vi "Hat Switch Interpreter.vi"(5 "JoystickDevRef":T1={"Device"=enum."USB 1"}) -> (0 "Buttons":bool[](array[boolean]), 1 "Buttons Pressed":bool[](array[boolean]), 2 "Enum Status":T4(ring), 3 "Numeric Status":u8, 4 "Hat Switch Cluster":T3)   [LabVIEW 2014]
uses:
  <vilib>/Rock Robotics/WPI/Joystick/WPI_JoystickDevRef.ctl
  <vilib>/Rock Robotics/WPI/Joystick/WPI_JoystickDeviceEnum.ctl
panel:
  # "ENUM LAYOUT"
  # "NUMERIC LAYOUT"
  # "North"
  # "1"
  # "Northeast"
  # "2"
  # "Northwest"
  # "8"
  # "West"
  # "East"
  # "7"
  # "3"
  # "Null"
  # "0"
  # "Southwest"
  # "Southeast"
  # "6"
  # "4"
  # "5"
  # "South"
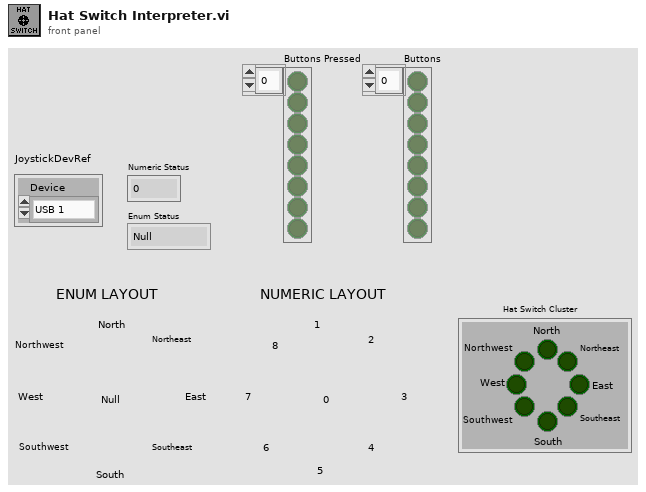
[diagram p1: front panel]
types:
  T1 = typedef "WPI_JoystickDevRef.ctl" = cluster{"Device":T2}
  T2 = typedef "WPI_JoystickDeviceEnum.ctl" = enum16{"USB 0", "USB 1", "USB 2", "USB 3", "USB 4", "USB 5"}
  T3 = cluster{"North":bool, "Northeast":bool, "East":bool, "Southeast":bool, "South":bool, "Southwest":bool, "West":bool, "Northwest":bool}
  T4 = enum8{"Null", "North", "Northeast", "East", "Southeast", "South", "Southwest", "West", "Northwest"}
  T5 = cluster{"North":bool, "Northeast":bool, "East":bool, "Southeast":bool, "South":bool, "Northwest":bool, "Southwest":bool, "West":bool}
  T6 = cluster{"[0]":bool, "[1]":bool, "[2]":bool, "[3]":bool, "[4]":bool, "[5]":bool, "[6]":bool, "[7]":bool, "[8]":bool}
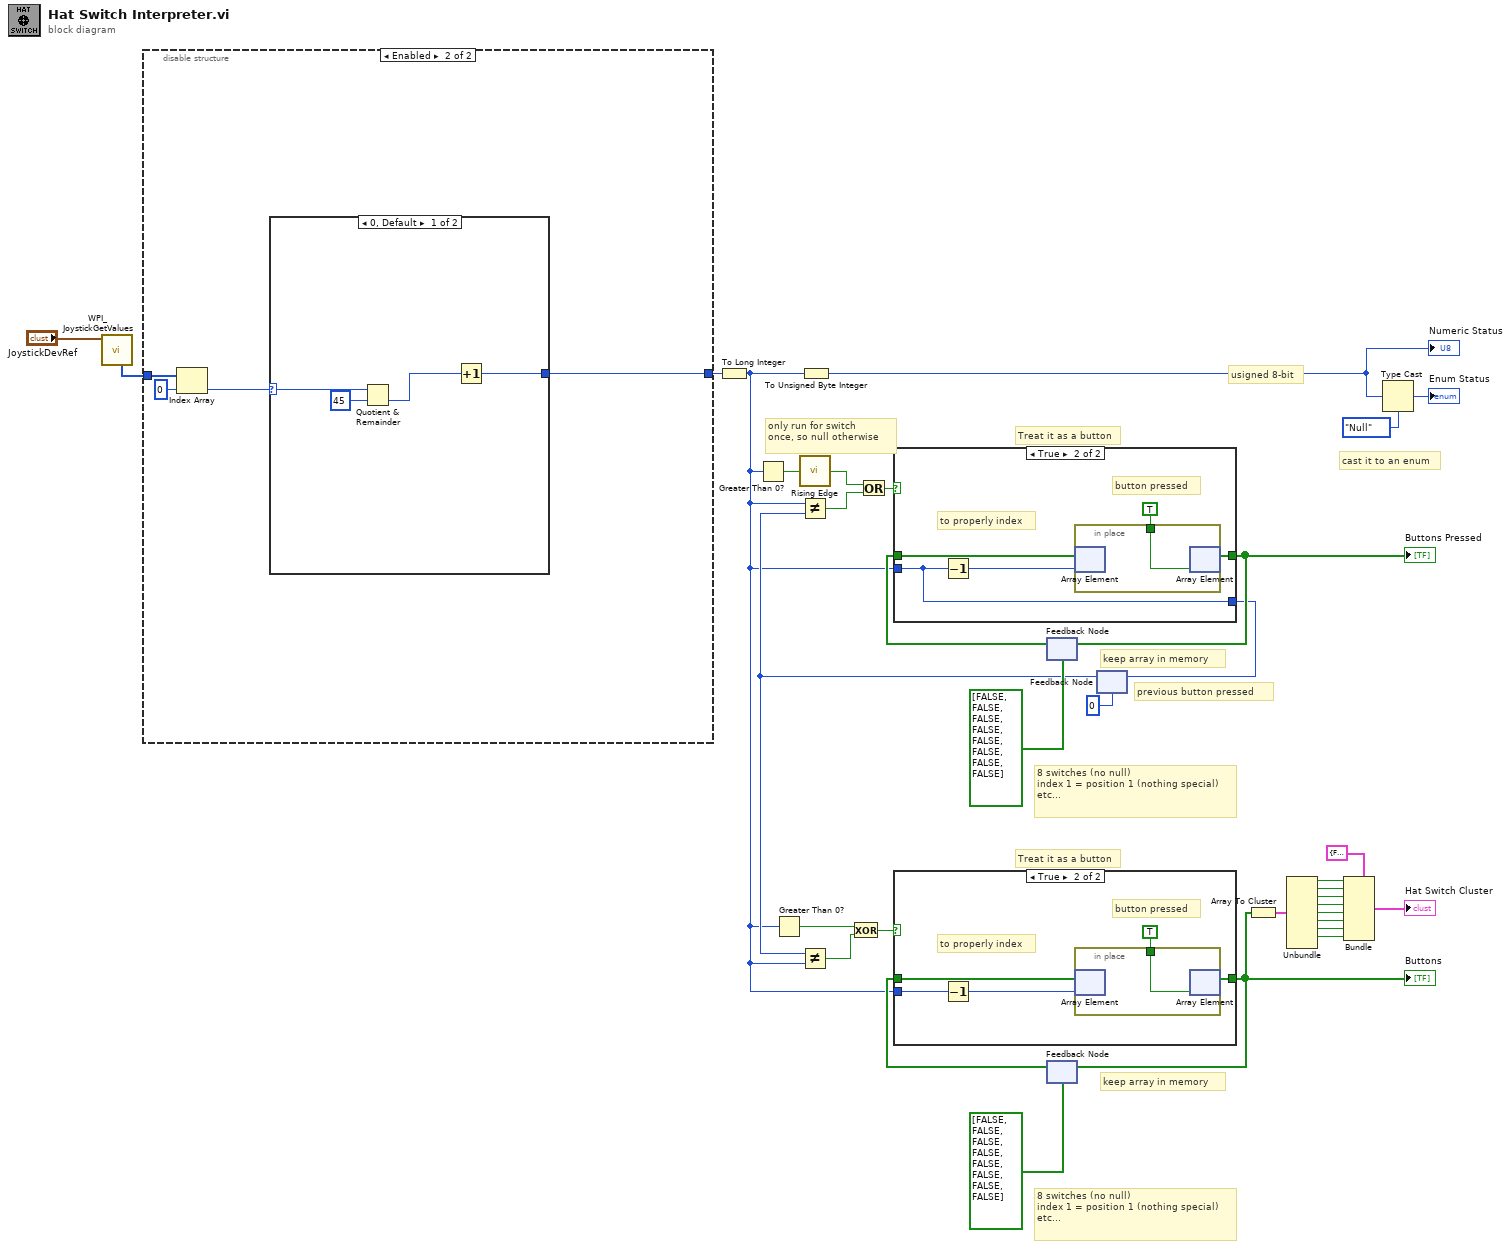
[diagram p0: block diagram]
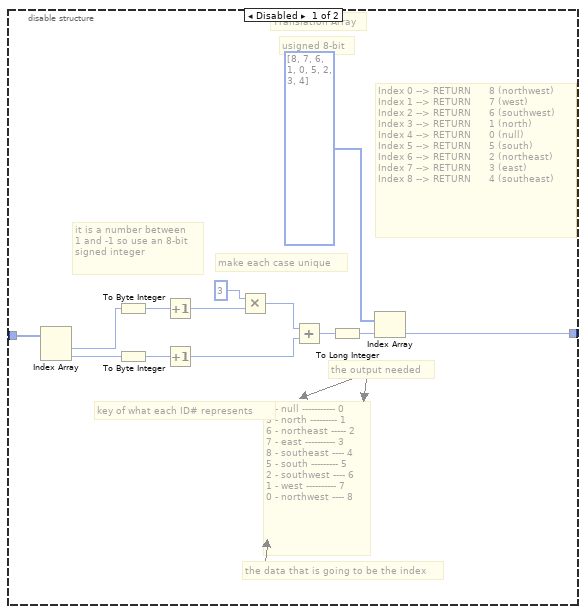
[diagram p2: hidden frame]
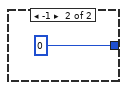
[diagram p3: hidden frame]
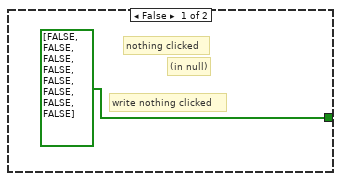
[diagram p4: hidden frame]
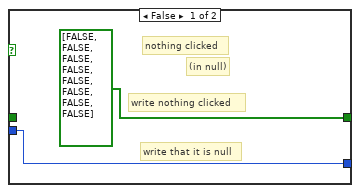
[diagram p5: hidden frame]
diagram:
  # "cast it to an enum"
  # "keep array in memory"
  # "8 switches (no null)\nindex 1 = position 1 (nothing special)\netc..."
  # "Treat it as a button"
  # "only run for switch\nonce, so null otherwise"
  # "keep array in memory"
  # "previous button pressed"
  # "8 switches (no null)\nindex 1 = position 1 (nothing special)\netc..."
  # "Treat it as a button"
  # "usigned 8-bit"
  n1 = call <vilib>:"WPI_JoystickGetValues.vi"("JoystickDevRef"="JoystickDevRef") -> ("POVs"=w4:i16[])  [unwired: 6 in, 4 out]
  n2 = disable-structure shown="Enabled" {
    disable-tunnel: [w38 w48] -> w26
    disable-tunnel: w4 -> [w37 w51]
    frame Disabled {
      # "usigned 8-bit"
      # "the data that is going to be the index"
      # "the output needed"
      # "key of what each ID# represents"
      # "Index 0 --> RETURN      8 (northwest)\nIndex 1 --> RETURN      7 (west)\nIndex 2 --> RETURN      6 (southwest)\nIndex 3 --> RETURN      1 (north)\nIndex 4 --> RETURN      0 (null)\nIndex 5 --> RETURN      5 (south)\nIndex 6 --> RETURN      2 (northeast)\nIndex 7 --> RETURN      3 (east)\nIndex 8 --> RETURN      4 (southeast)"
      # "4 - null ----------- 0\n3 - north --------- 1\n6 - northeast ----- 2\n7 - east ---------- 3\n8 - southeast ---- 4\n5 - south --------- 5\n2 - southwest ---- 6\n1 - west ---------- 7\n0 - northwest ---- 8"
      # "Translation Array"
      # "it is a number between\n1 and -1 so use an 8-bit\nsigned integer"
      # "make each case unique"
      n3 = Index Array(array=w37) -> (element #1=w36:i16, element #2=w35:i16)  [unwired: 2 in]
      n4 = To Byte Integer(number=w36) -> (8bit integer=w43:i8)
      n5 = To Byte Integer(number=w35) -> (8bit integer=w42:i8)
      n6 = Increment(x=w43) -> (x+1=w47:i8)
      n7 = Increment(x=w42) -> (x+1=w44:i8)
      n8 = Multiply(x=i8 3, y=w47) -> (x*y=w45:i8)
      n9 = Add(x=w45, y=w44) -> (x+y=w40:i8)
      n10 = To Long Integer(number=w40) -> (32bit integer=w39:i32)
      n11 = Index Array(array=u8[] [8, 7, 6, 1, 0, 5, 2, 3, 4], index=w39) -> (element=w38:u8)
    }
    frame Enabled {
      n12 = Index Array(array=w51, index=0) -> (element=w49:i16)
      n13 = case shown="0, Default" w49 {
        selector: w49 -> [w55 _]
        tunnel: [w52 i16 0] -> w48
        frame 0, Default {
          n14 = Quotient & Remainder(x=w55, y=i16 45) -> (floor(x/y)=w53:i16)  [unwired: 1 out]
          n15 = Increment(x=w53) -> (x+1=w52:i16)
        }
        frame -1 {
        }
      }
    }
  }
  n16 = To Long Integer(number=w26) -> (32bit integer=w20:i32)
  n17 = Greater Than 0?(x=w20) -> (x > 0?=w29:bool)
  n18 = Greater Than 0?(x=w20) -> (x > 0?=w22:bool)
  n19 = call "Rising Edge.vi"("Input"=w29) -> ("Rising Edge"=w28:bool)
  n20 = To Unsigned Byte Integer(number=w20) -> (unsigned 8bit integer=w3:u8)
  "Numeric Status" <- w3
  n21 = feedback #1(bool[] [FALSE, FALSE, FALSE, FALSE, FALSE, FALSE, FALSE, FALSE]) -> (w33:bool[])
  n22 = feedback #2(bool[] [FALSE, FALSE, FALSE, FALSE, FALSE, FALSE, FALSE, FALSE]) -> (w24:bool[])
  n23 = feedback #3(0) -> (w21:i32)
  n24 = Not Equal?(x=w20, y=w21) -> (x != y?=w25:bool)
  n25 = Not Equal?(x=w21, y=w20) -> (x != y?=w18:bool)
  n26 = Exclusive Or(1:w18, 2:w22) -> (0:w19:bool)
  n27 = Or(x=w28, y=w25) -> (x .or. y?=w27:bool)
  n28 = case shown="True" w27 {
    tunnel: w33 -> [_ w63]
    tunnel: [bool[] [FALSE, FALSE, FALSE, FALSE, FALSE, FALSE, FALSE, FALSE] w62] -> w32
    tunnel: w20 -> [w58 w59]
    tunnel: [w58 w59] -> w30
    frame False {
      # "write nothing clicked"
      # "write that it is null"
      # "(in null)"
      # "nothing clicked"
    }
    frame True {
      # "to properly index"
      # "button pressed"
      n29 = Decrement(x=w59) -> (x-1=w60:i32)
      n30 = in-place {
        in-place-border: TRUE -> [w64]
        n31 = in-place-array #4(w63, w60) -> ()  [unwired: 1 out]
        n32 = in-place-array #4(w64) -> (w62:bool[])  [unwired: 1 out]
      }
    }
  }
  "Buttons Pressed" <- w32
  n33 = case shown="True" w19 {
    tunnel: w24 -> [_ w70]
    tunnel: [bool[] [FALSE, FALSE, FALSE, FALSE, FALSE, FALSE, FALSE, FALSE] w69] -> w17
    tunnel: w20 -> [_ w66]
    frame False {
      # "write nothing clicked"
      # "(in null)"
      # "nothing clicked"
    }
    frame True {
      # "to properly index"
      # "button pressed"
      n34 = Decrement(x=w66) -> (x-1=w67:i32)
      n35 = in-place {
        in-place-border: TRUE -> [w71]
        n36 = in-place-array #5(w70, w67) -> ()  [unwired: 1 out]
        n37 = in-place-array #5(w71) -> (w69:bool[])  [unwired: 1 out]
      }
    }
  }
  "Buttons" <- w17
  n38 = feedback-in #1(w32) -> ()
  n39 = feedback-in #2(w17) -> ()
  n40 = feedback-in #3(w30) -> ()
  n41 = Array To Cluster(array=w17) -> (cluster=w16:T6)
  n42 = Unbundle(w16) -> ("[0]"=w14:bool, "[1]"=w6:bool, "[2]"=w7:bool, "[3]"=w8:bool, "[4]"=w9:bool, "[5]"=w10:bool, "[6]"=w11:bool, "[7]"=w12:bool)  [unwired: 1 out]
  n43 = Bundle(cluster=T5 {"North"=FALSE, "Northeast"=FALSE, "East"=FALSE, "Southeast"=FALSE, "South"=FALSE, "Northwest"=FALSE, "Southwest"=FALSE, "West"=FALSE} ("Hat Switch Cluster"), "North"=w14, "Northeast"=w6, "East"=w7, "Southeast"=w8, "South"=w9, "Northwest"=w10, "Southwest"=w11, "West"=w12) -> (→"Hat Switch Cluster":T5)
  n44 = Type Cast(type=T4."Null" ("Enum Status"), x=w3) -> (*(type *) &x=→"Enum Status":T4)
